vi "Save File WILT Open Close Save References.vi"(4 "Save Data":string[](array[string]), 6 "New File?":bool, 8 "error in (no error)":errorcluster, 9 "File Path Output New in":T1, 10 "Status Color":u32(colorbox), 11 "Byte Stream File in":refnum<file>) -> (0 "error out":errorcluster, 1 "First Time Through Out":bool, 2 "File Path Output New out":T1, 3 "Byte Stream File out":refnum<file>)   [LabVIEW 2016, in "Save File.lvlib"]
uses:
  Save File.lvlib
  File Setup (Public)/Type Definition/Save File DOE File Path Control.ctl
  File Setup (Public)/Type Definition/Save File DOE Data Save Filepaths.ctl
  File Setup.lvlib
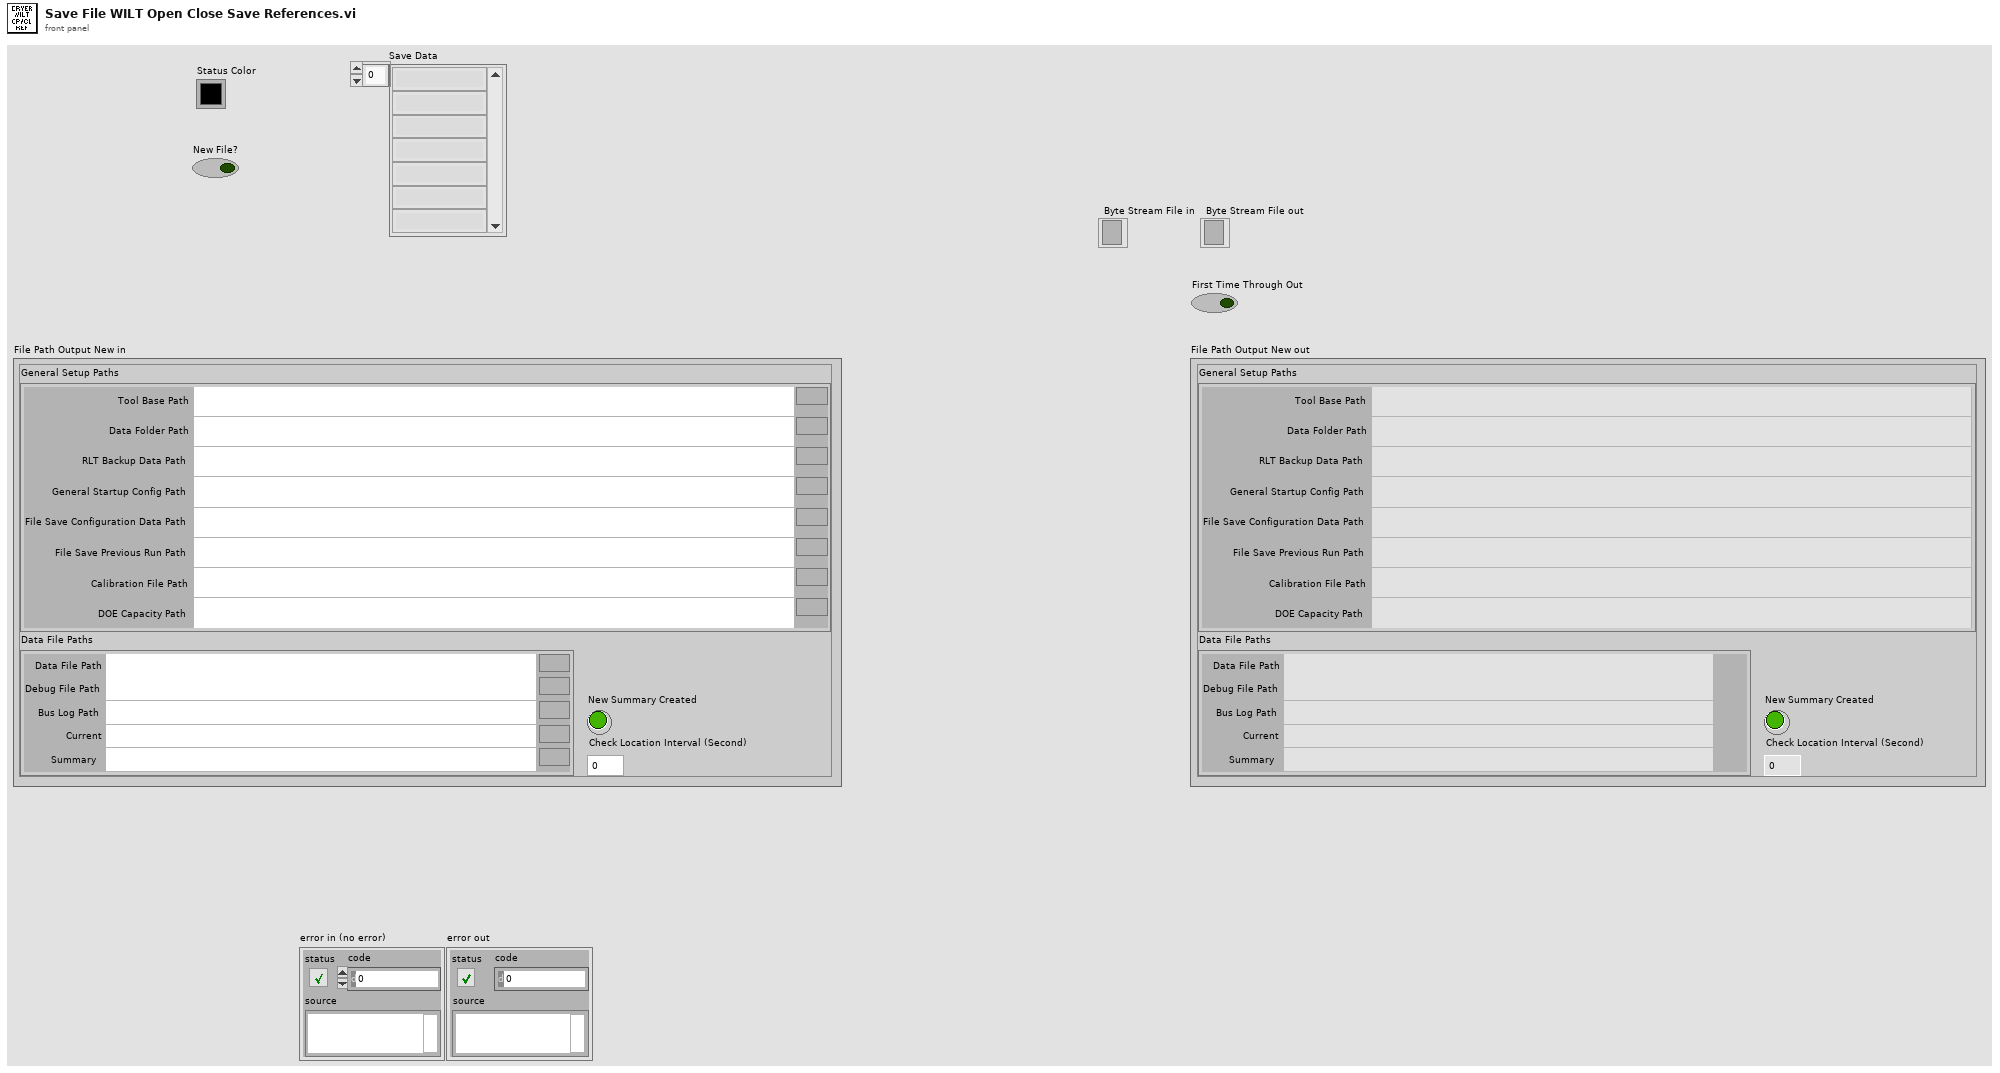
[diagram p1: front panel]
types:
  T1 = typedef "File Setup.lvlib/Save File DOE File Path Control.ctl" = cluster{"General Setup Paths":cluster{"Calibration File Path":path, "DOE Capacity Path":path, "Data Folder Path":path, "RLT Backup Data Path":path, "Tool Base Path":path, "General Startup Config Path":path, "File Save Previous Run Path":path, "File Save Configuration Data Path":path}, "Data File Paths":T2, "New Summary Created":bool, "Check Location Interval (Second)":i32}
  T2 = typedef "File Setup.lvlib/Save File DOE Data Save Filepaths.ctl" = cluster{"Data File Path":path, "Debug File Path":path, "Bus Log Path":path, "Current":path, "Summary":path}
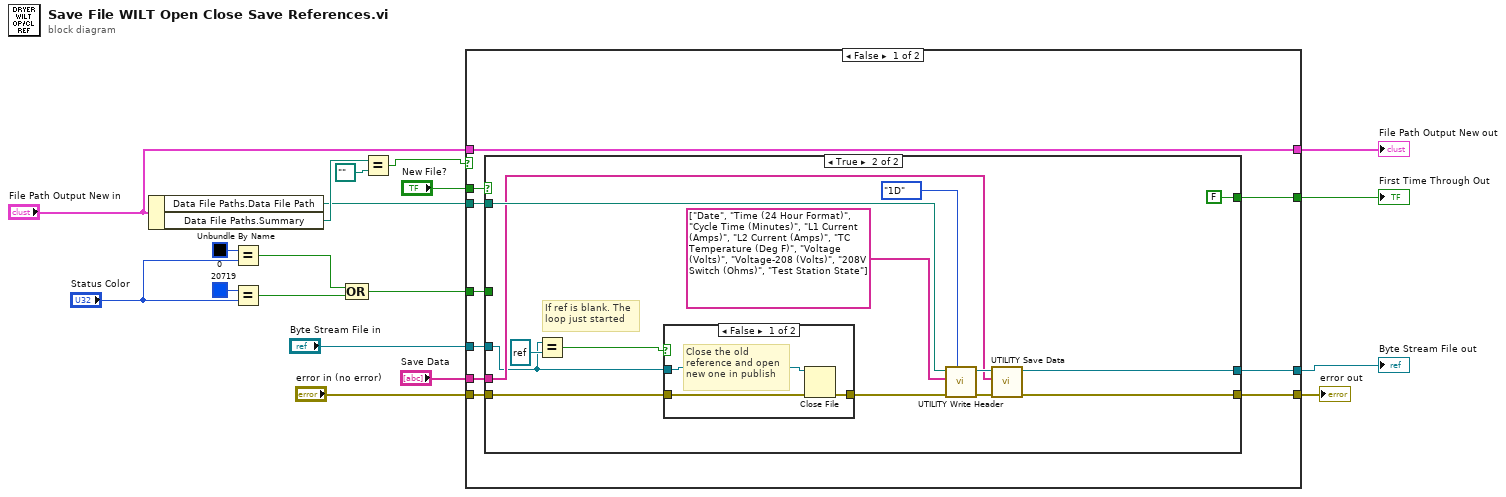
[diagram p0: block diagram]
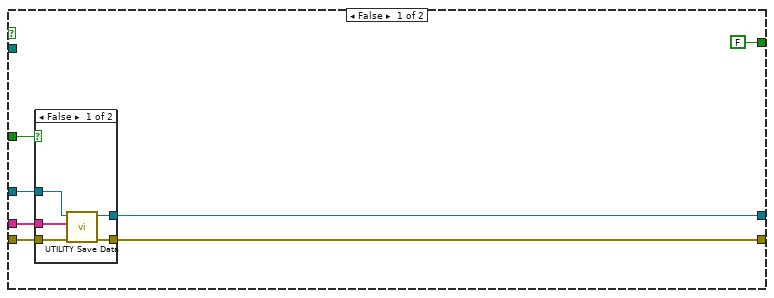
[diagram p2: hidden frame]
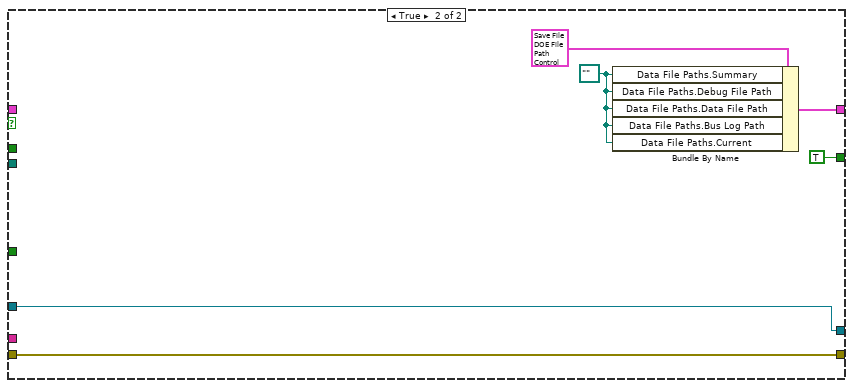
[diagram p5: hidden frame]
diagram:
  n1 = Unbundle By Name("File Path Output New in") -> ("Data File Paths.Data File Path"=w8:path, "Data File Paths.Summary"=w11:path)
  n2 = Equal?(x=u32 0 ("Startup"), y="Status Color") -> (x = y?=w6:bool)
  n3 = Equal?(x=u32 20719 ("EOC"), y="Status Color") -> (x = y?=w7:bool)
  n4 = Compound Arithmetic op=OR(w6, w7) -> (w5:bool)
  n5 = Equal?(x=w11, y=path "") -> (x = y?=w1:bool)
  n6 = case shown="False" w1 {
    tunnel: "New File?" -> [w29 _]
    tunnel: [w28 TRUE] -> w13
    tunnel: "Save Data" -> [w27 _]
    tunnel: "File Path Output New in" -> [w26 _]
    tunnel: [w26 w65] -> w15
    tunnel: w5 -> [w25 _]
    tunnel: [w24 w63] -> w16
    tunnel: "Byte Stream File in" -> [w23 w63]
    tunnel: "error in (no error)" -> [w22 w62]
    tunnel: [w21 w62] -> w19
    tunnel: w8 -> [w20 _]
    frame False {
      n7 = case shown="True" w29 {
        tunnel: w20 -> [_ w53]
        tunnel: w27 -> [w36 w52]
        tunnel: [FALSE FALSE] -> w28
        tunnel: w25 -> [w34 _]
        tunnel: [w32 w51] -> w24
        tunnel: w23 -> [w33 w48]
        tunnel: w22 -> [w31 w47]
        tunnel: [w30 w45] -> w21
        frame False {
          n8 = case shown="False" w34 {
            tunnel: w36 -> [w40 _]
            tunnel: w33 -> [w41 w43]
            tunnel: [w39 w43] -> w32
            tunnel: w31 -> [w38 w42]
            tunnel: [w37 w42] -> w30
            frame False {
              n9 = call "UTILITY Save Data.vi"("error in"=w38, "Data"=w40, "refnum"=w41) -> ("error out"=w37:errorcluster, "refnum out"=w39:refnum<file>)  [unwired: 7 in]
            }
            frame True {
            }
          }
        }
        frame True {
          # "If ref is blank. The\nloop just started"
          n10 = Equal?(x=w48, y=refnum<file> refnum ("Blank")) -> (x = y?=w49:bool)
          n11 = case shown="False" w49 {
            tunnel: w48 -> [w60 _]
            tunnel: w47 -> [w59 w61]
            tunnel: [w58 w61] -> w46
            frame False {
              # "Close the old\nreference and open\nnew one in publish"
              n12 = Close File(refnum=w60, error in=w59) -> (error out=w58:errorcluster)  [unwired: 1 out]
            }
            frame True {
            }
          }
          n13 = call "UTILITY Write Header.vi"("Array Type"=enum16{"1D", "2D"}."1D", "error in (no error)"=w46, "Headers"=string[] ["Date", "Time (24 Hour Format)", "Cycle Time (Minutes)", "L1 Current (Amps)", "L2 Current (Amps)", "TC Temperature (Deg F)", "Voltage (Volts)", "Voltage-208 (Volts)", "208V Switch (Ohms)", "Test Station State"], "File Path Control"=w53) -> ("error out"=w56:errorcluster, "Byte Stream File out"=w55:refnum<file>)  [unwired: 6 in]
          n14 = call "UTILITY Save Data.vi"("error in"=w56, "Data"=w52, "refnum"=w55) -> ("error out"=w45:errorcluster, "refnum out"=w51:refnum<file>)  [unwired: 7 in]
        }
      }
    }
    frame True {
      w64 = path "" ("Log Debug File")
      n15 = Bundle By Name(cluster=T1 {"General Setup Paths"={"Calibration File Path"=path "", "DOE Capacity Path"=path "", "Data Folder Path"=path "", "RLT Backup Data Path"=path "", "Tool Base Path"=path "", "General Startup Config Path"=path "", "File Save Previous Run Path"=path "", "File Save Configuration Data Path"=path ""}, "Data File Paths"={"Data File Path"=path "", "Debug File Path"=path "", "Bus Log Path"=path "", "Current"=path "", "Summary"=path ""}, "New Summary Created"=FALSE, "Check Location Interval (Second)"=0} ("File Path Output New"), "Data File Paths.Summary"=w64, "Data File Paths.Debug File Path"=w64, "Data File Paths.Data File Path"=w64, "Data File Paths.Bus Log Path"=w64, "Data File Paths.Current"=w64) -> (w65:T1)
    }
  }
  "error out" <- w19
  "Byte Stream File out" <- w16
  "File Path Output New out" <- w15
  "First Time Through Out" <- w13
